vi "S2DS_Core decision-New.vi"(6 "Ramp X":bool, 7 "Ramp Y":bool, 9 "Scan parameters out  in":T1 {"Y data taking" items=["in both direction", "in up direction only", "in down direction only"]; "X data taking" items=["in both direction", "in up direction only", "in down direction only"]}, 10 "Sweep ON?":bool) -> (1 "Turn off Sweep?":bool, 2 "Sweep Over?":bool, 3 "Scan parameters out":T1 {"Y data taking" items=["in both direction", "in up direction only", "in down direction only"]; "X data taking" items=["in both direction", "in up direction only", "in down direction only"]})   [LabVIEW 2025]
uses:
  TYPE DEFS/S2DS_Sweep Info.ctl
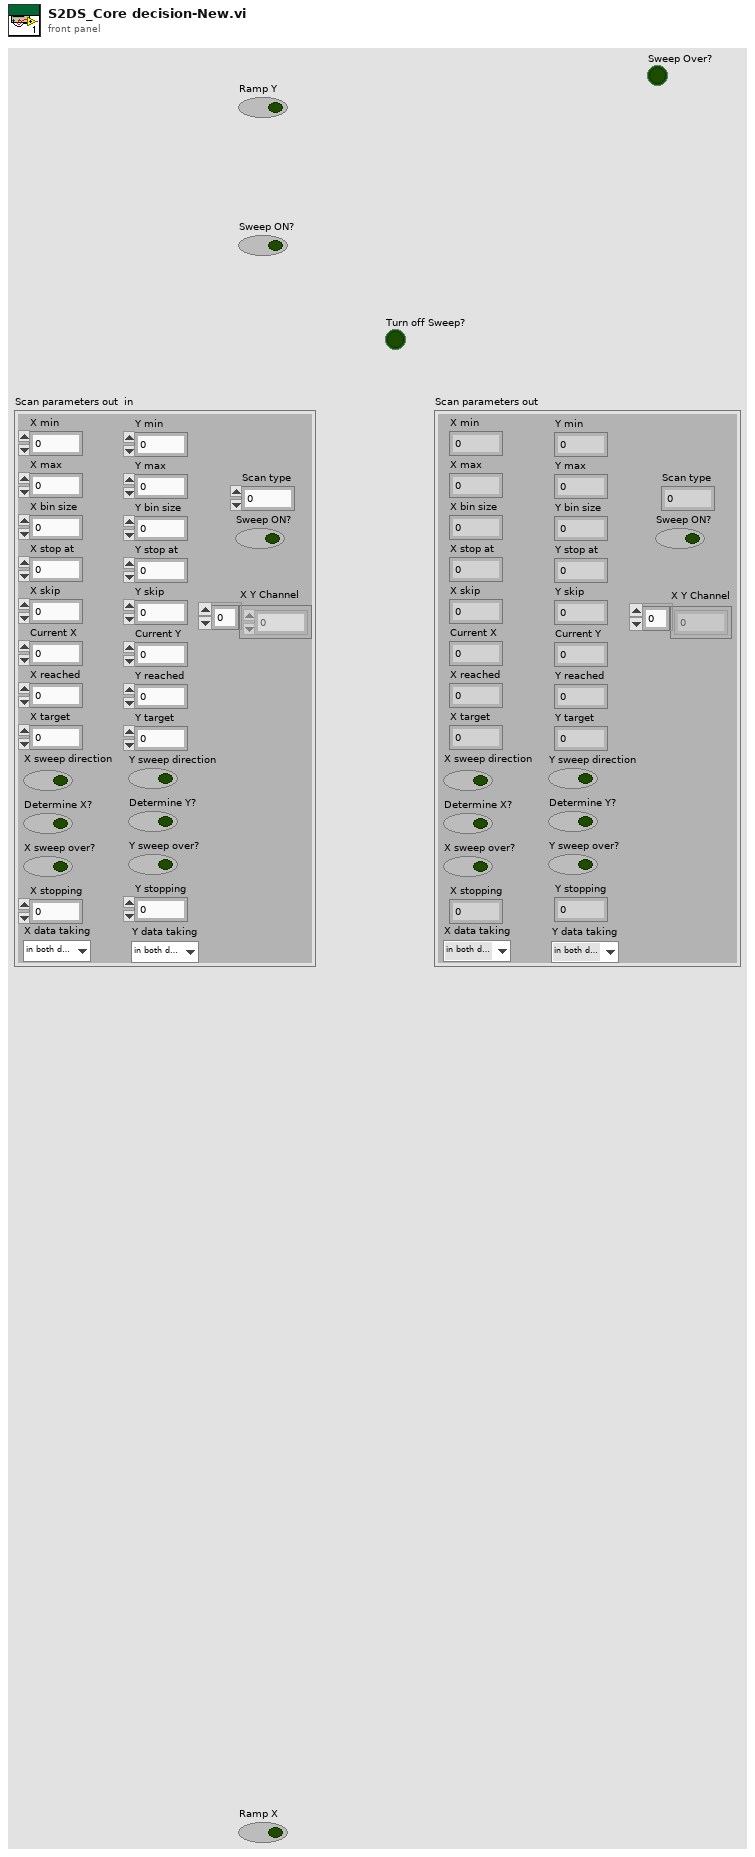
[diagram p1: front panel]
types:
  T1 = typedef "S2DS_Sweep Info.ctl" = cluster{"X min":ext, "X max":dbl, "Y min":dbl, "Y max":dbl, "X bin size":dbl, "Y bin size":dbl, "X stop at":dbl, "Y stop at":dbl, "X skip":u64, "Y skip":u64, "Current X":dbl, "Current Y":dbl, "X reached":i32, "Y reached":i32, "X target":dbl, "Y target":dbl, "Sweep ON?":bool, "X sweep direction":bool, "Y sweep direction":bool, "Determine X?":bool, "Determine Y?":bool, "X sweep over?":bool, "Y sweep over?":bool, "Scan type":i32, "X stopping":i32, "Y stopping":i32, "X Y Channel":u16[], "X data taking":u16, "Y data taking":u16}
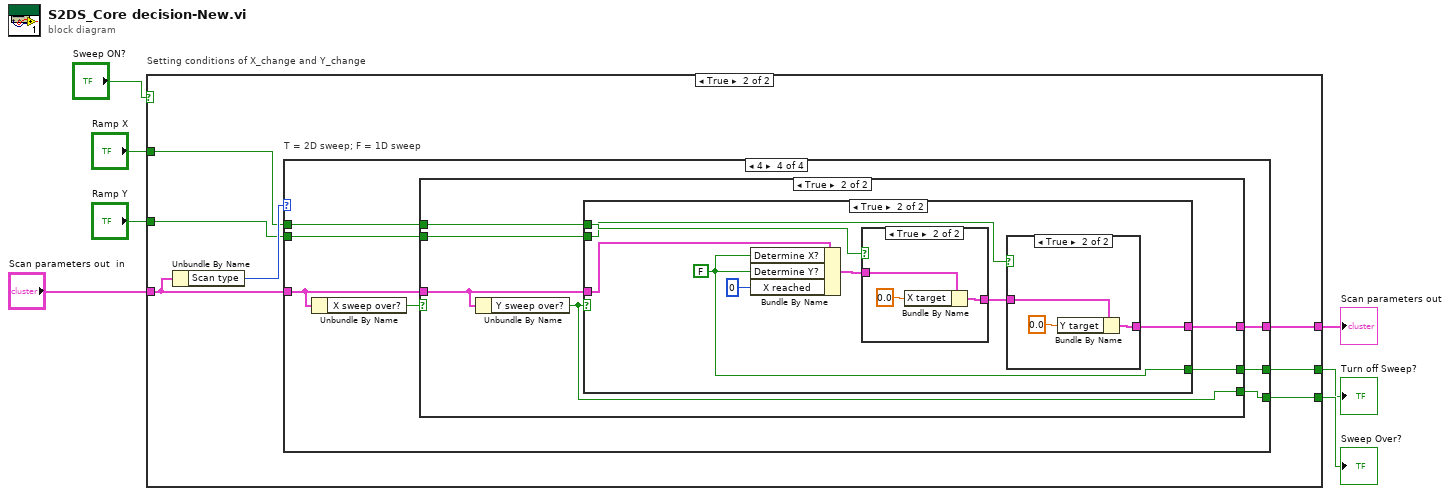
[diagram p0: block diagram]
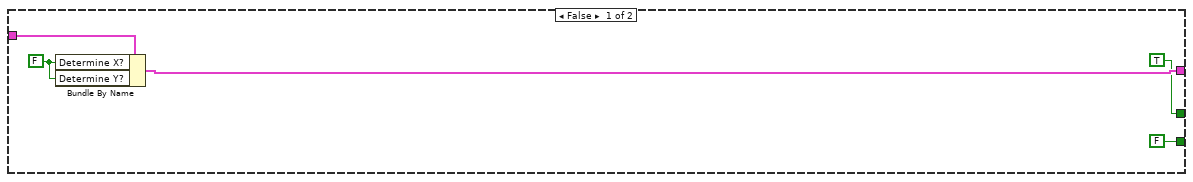
[diagram p2: hidden frame]
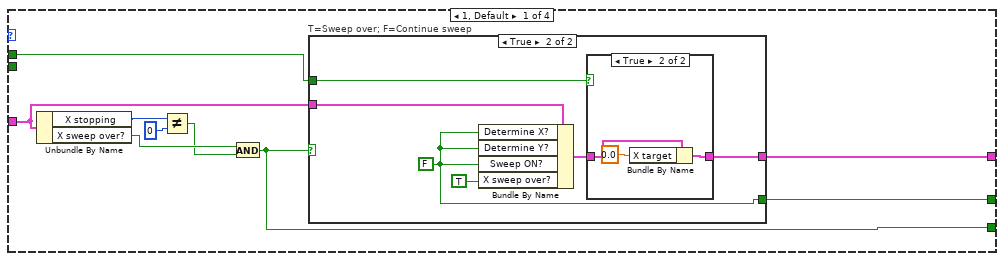
[diagram p3: hidden frame]
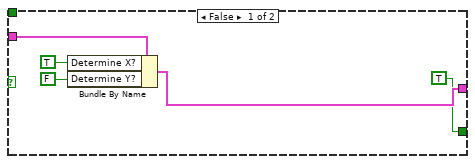
[diagram p4: hidden frame]
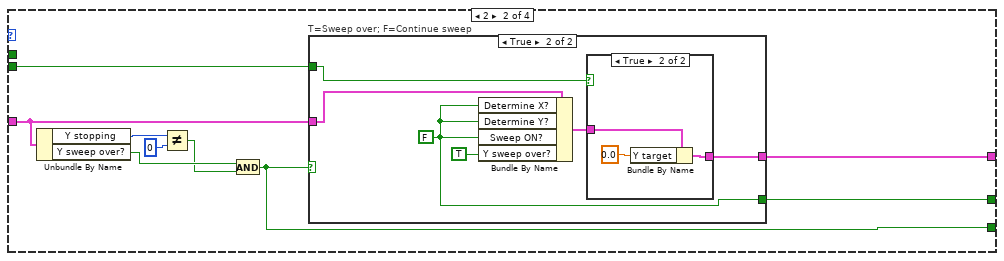
[diagram p6: hidden frame]
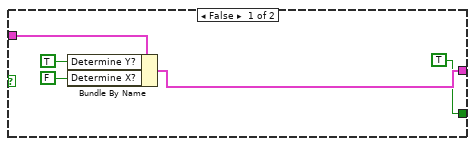
[diagram p7: hidden frame]
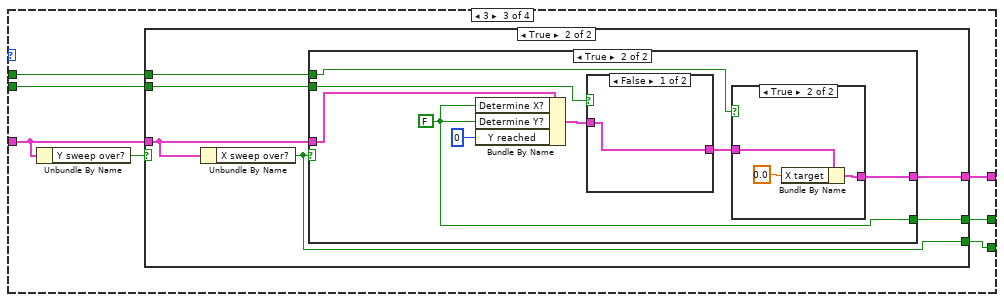
[diagram p9: hidden frame]
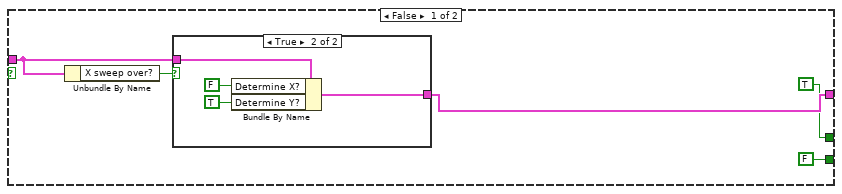
[diagram p10: hidden frame]
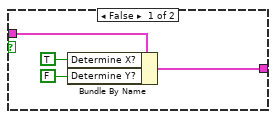
[diagram p11: hidden frame]
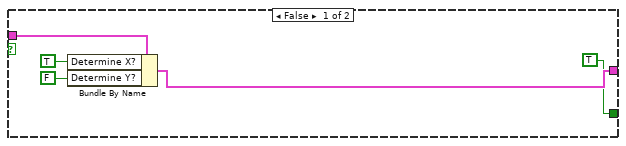
[diagram p12: hidden frame]
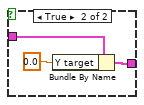
[diagram p14: hidden frame]
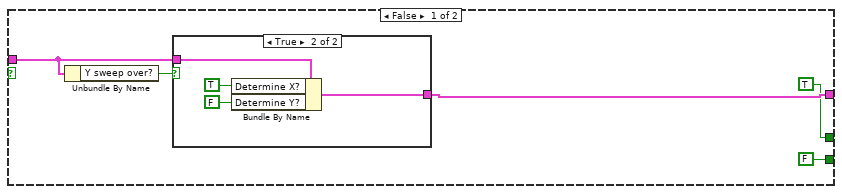
[diagram p15: hidden frame]
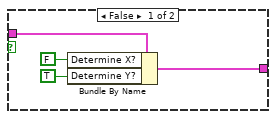
[diagram p16: hidden frame]
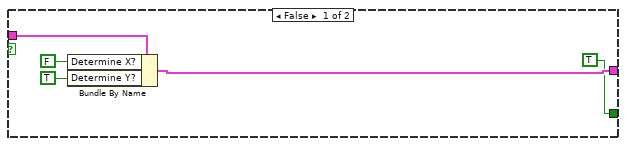
[diagram p17: hidden frame]
diagram:
  n1 = case "Setting conditions of X_change and Y_change" shown="True" "Sweep ON?" {
    tunnel: "Scan parameters out  in" -> [w12 w19]
    tunnel: [w10 w18] -> w3
    tunnel: "Ramp X" -> [_ w16]
    tunnel: "Ramp Y" -> [_ w15]
    tunnel: [FALSE ("Y sweep over?") w14] -> w2
    tunnel: [TRUE ("Change X?") w13] -> w1
    frame False {
      w11 = FALSE
      n2 = Bundle By Name(cluster=w12, "Determine X?"=w11, "Determine Y?"=w11) -> (w10:T1)
    }
    frame True {
      n3 = Unbundle By Name(w19) -> ("Scan type"=w17:i32)
      n4 = case "T = 2D sweep; F = 1D sweep" shown="4" w17 {
        tunnel: w19 -> [w27 w51 w73 w120]
        tunnel: [w26 w50 w72 w119] -> w18
        tunnel: w16 -> [w22 _ w70 w118]
        tunnel: w15 -> [_ w46 w71 w117]
        tunnel: [w21 w45 w69 w116] -> w14
        tunnel: [w20 w44 w68 w115] -> w13
        frame 1, Default {
          n5 = Unbundle By Name(w27) -> ("X stopping"=w23:i32, "X sweep over?"=w28:bool)
          n6 = Not Equal?(x=w23, y=0) -> (x != y?=w24:bool)
          n7 = And(x=w28, y=w24) -> (x .and. y?=w21:bool)
          n8 = case "T=Sweep over; F=Continue sweep" shown="True" w21 {
            tunnel: w27 -> [w31 w39]
            tunnel: [w30 w36] -> w26
            tunnel: w22 -> [_ w35]
            tunnel: [TRUE ("Change X?") w34] -> w20
            frame False {
              n9 = Bundle By Name(cluster=w31, "Determine X?"=TRUE ("Change X?"), "Determine Y?"=FALSE ("Change X?")) -> (w30:T1)
            }
            frame True {
              w34 = FALSE ("Change X?")
              n10 = Bundle By Name(cluster=w39, "Determine X?"=w34, "Determine Y?"=w34, "Sweep ON?"=w34, "X sweep over?"=TRUE) -> (w37:T1)
              n11 = case shown="True" w35 {
                tunnel: w37 -> [w40 w43]
                tunnel: [w40 w41] -> w36
                frame False {
                }
                frame True {
                  n12 = Bundle By Name(cluster=w43, "X target"=0.0) -> (w41:T1)
                }
              }
            }
          }
        }
        frame 2 {
          n13 = Unbundle By Name(w51) -> ("Y stopping"=w47:i32, "Y sweep over?"=w52:bool)
          n14 = Not Equal?(x=w47, y=0) -> (x != y?=w48:bool)
          n15 = And(x=w52, y=w48) -> (x .and. y?=w45:bool)
          n16 = case "T=Sweep over; F=Continue sweep" shown="True" w45 {
            tunnel: w51 -> [w55 w63]
            tunnel: [w54 w59] -> w50
            tunnel: w46 -> [_ w61]
            tunnel: [TRUE ("Change X?") w58] -> w44
            frame False {
              n17 = Bundle By Name(cluster=w55, "Determine Y?"=TRUE ("Change X?"), "Determine X?"=FALSE ("Change X?")) -> (w54:T1)
            }
            frame True {
              w58 = FALSE ("Change X?")
              n18 = Bundle By Name(cluster=w63, "Determine X?"=w58, "Determine Y?"=w58, "Sweep ON?"=w58, "Y sweep over?"=TRUE) -> (w60:T1)
              n19 = case shown="True" w61 {
                tunnel: w60 -> [w64 w67]
                tunnel: [w64 w65] -> w59
                frame False {
                }
                frame True {
                  n20 = Bundle By Name(cluster=w67, "Y target"=0.0) -> (w65:T1)
                }
              }
            }
          }
        }
        frame 3 {
          n21 = Unbundle By Name(w73) -> ("Y sweep over?"=w74:bool)
          n22 = case shown="True" w74 {
            tunnel: w73 -> [w78 w92]
            tunnel: [w77 w93] -> w72
            tunnel: w71 -> [_ w91]
            tunnel: w70 -> [_ w90]
            tunnel: [FALSE ("X sweep over?") w89] -> w69
            tunnel: [TRUE w88] -> w68
            frame False {
              n23 = Unbundle By Name(w78) -> ("X sweep over?"=w79:bool)
              n24 = case shown="True" w79 {
                tunnel: w78 -> [w83 w87]
                tunnel: [w82 w86] -> w77
                frame False {
                  n25 = Bundle By Name(cluster=w83, "Determine X?"=TRUE, "Determine Y?"=FALSE) -> (w82:T1)
                }
                frame True {
                  n26 = Bundle By Name(cluster=w87, "Determine X?"=FALSE, "Determine Y?"=TRUE) -> (w86:T1)
                }
              }
            }
            frame True {
              n27 = Unbundle By Name(w92) -> ("X sweep over?"=w89:bool)
              n28 = case shown="True" w89 {
                tunnel: w92 -> [w95 w106]
                tunnel: [w96 w101] -> w93
                tunnel: w91 -> [_ w103]
                tunnel: w90 -> [_ w100]
                tunnel: [TRUE w99] -> w88
                frame False {
                  n29 = Bundle By Name(cluster=w95, "Determine X?"=TRUE, "Determine Y?"=FALSE) -> (w96:T1)
                }
                frame True {
                  w99 = FALSE
                  n30 = Bundle By Name(cluster=w106, "Determine X?"=w99, "Determine Y?"=w99, "Y reached"=0) -> (w104:T1)
                  n31 = case shown="False" w103 {
                    tunnel: w104 -> [w111 w114]
                    tunnel: [w111 w112] -> w102
                    frame False {
                    }
                    frame True {
                      n32 = Bundle By Name(cluster=w114, "Y target"=0.0) -> (w112:T1)
                    }
                  }
                  n33 = case shown="True" w100 {
                    tunnel: w102 -> [w107 w110]
                    tunnel: [w107 w108] -> w101
                    frame False {
                    }
                    frame True {
                      n34 = Bundle By Name(cluster=w110, "X target"=0.0) -> (w108:T1)
                    }
                  }
                }
              }
            }
          }
        }
        frame 4 {
          n35 = Unbundle By Name(w120) -> ("X sweep over?"=w121:bool)
          n36 = case shown="True" w121 {
            tunnel: w120 -> [w125 w139]
            tunnel: [w124 w140] -> w119
            tunnel: w118 -> [_ w138]
            tunnel: w117 -> [_ w137]
            tunnel: [FALSE ("Y sweep over?") w136] -> w116
            tunnel: [TRUE w135] -> w115
            frame False {
              n37 = Unbundle By Name(w125) -> ("Y sweep over?"=w126:bool)
              n38 = case shown="True" w126 {
                tunnel: w125 -> [w130 w134]
                tunnel: [w129 w133] -> w124
                frame False {
                  n39 = Bundle By Name(cluster=w130, "Determine X?"=FALSE, "Determine Y?"=TRUE) -> (w129:T1)
                }
                frame True {
                  n40 = Bundle By Name(cluster=w134, "Determine X?"=TRUE, "Determine Y?"=FALSE) -> (w133:T1)
                }
              }
            }
            frame True {
              n41 = Unbundle By Name(w139) -> ("Y sweep over?"=w136:bool)
              n42 = case shown="True" w136 {
                tunnel: w139 -> [w142 w153]
                tunnel: [w143 w149] -> w140
                tunnel: w138 -> [_ w148]
                tunnel: w137 -> [_ w147]
                tunnel: [TRUE w146] -> w135
                frame False {
                  n43 = Bundle By Name(cluster=w142, "Determine X?"=FALSE, "Determine Y?"=TRUE) -> (w143:T1)
                }
                frame True {
                  w146 = FALSE
                  n44 = Bundle By Name(cluster=w153, "Determine X?"=w146, "Determine Y?"=w146, "X reached"=0) -> (w151:T1)
                  n45 = case shown="True" w148 {
                    tunnel: w151 -> [w158 w161]
                    tunnel: [w158 w159] -> w150
                    frame False {
                    }
                    frame True {
                      n46 = Bundle By Name(cluster=w161, "X target"=0.0) -> (w159:T1)
                    }
                  }
                  n47 = case shown="True" w147 {
                    tunnel: w150 -> [w154 w157]
                    tunnel: [w154 w155] -> w149
                    frame False {
                    }
                    frame True {
                      n48 = Bundle By Name(cluster=w157, "Y target"=0.0) -> (w155:T1)
                    }
                  }
                }
              }
            }
          }
        }
      }
    }
  }
  "Scan parameters out" <- w3
  "Sweep Over?" <- w2
  "Turn off Sweep?" <- w1
